vi "Write Temp YAML File.vi"(8 "Error In":errorcluster) -> (0 "Error Out":errorcluster)   [LabVIEW 2010]
panel:
  in  "Provenance":cluster{"filename":string, "software":string}={"filename"="File Name", "software"="Acquisition Software"}
  in  "Identity":T1={"author"="Author Name", "author_affiliation"="Company Name"}
  in  "Sample":T2={"sample_name"="Sample Name", "buffer_name"="Buffer Name", "dye_names"="Cy3B, ATTO647N"}
  in  "Description":string="this is a description"
  in  "Photon Data":T3={"Time Stamp Unit"=1e-08, "Measurement Type"=enum."smFRET", "Spectral Channels List"=[{"Detector IDs"=[0]}, {"Detector IDs"=[1]}]}
  in  "Excitation Types":bool[](array[boolean])=[FALSE]
  in  "detection_wavelengths":dbl[unit][](array[numeric])=[5.800000000000001e-07, 6.4e-07] caption="Detection Wavelengths"
  in  "excitation_wavelengths":dbl[unit][](array[numeric])=[5.32e-07] caption="Excitation Wavelengths"
  in  "Setup (Mandatory)":T4={"num_pixels"=2, "num_spots"=1, "num_spectral_ch"=2, "num_polarization_ch"=1, "num_split_ch"=1, "modulated_excitation"=FALSE, "lifetime"=FALSE}
  # "Photon Data"
  # "Setup (Optional)"
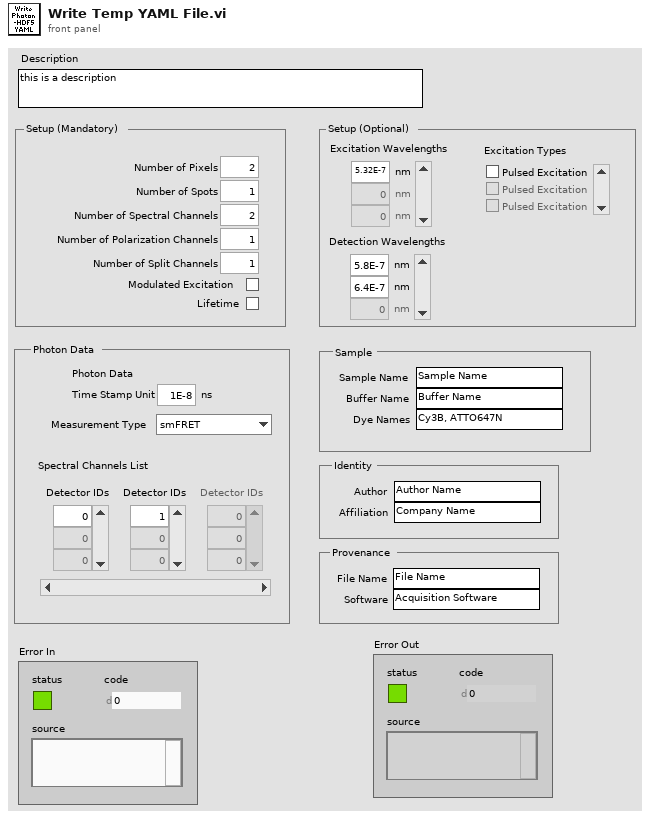
[diagram p1: front panel]
types:
  T1 = cluster{"author":string, "author_affiliation":string}
  T2 = cluster{"sample_name":string, "buffer_name":string, "dye_names":string}
  T3 = cluster{"Time Stamp Unit":dbl[unit], "Measurement Type":enum16{"Undefined", "smFRET"}, "Spectral Channels List":cluster{"Detector IDs":u8[]}[]}
  T4 = cluster{"num_pixels":u8, "num_spots":u8, "num_spectral_ch":u8, "num_polarization_ch":u8, "num_split_ch":u8, "modulated_excitation":bool, "lifetime":bool}
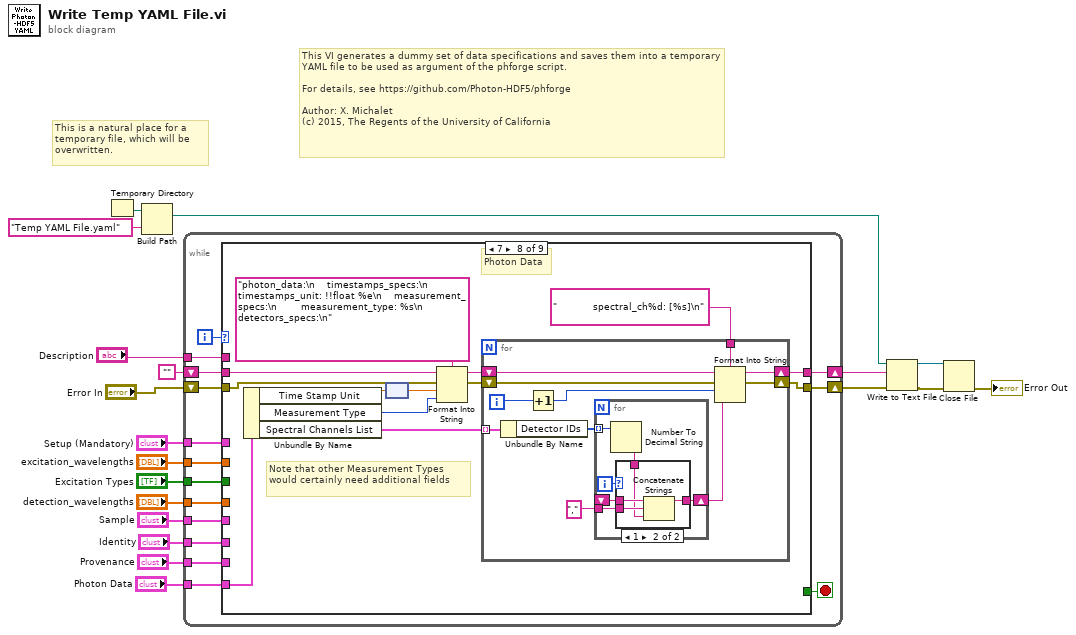
[diagram p0: block diagram]
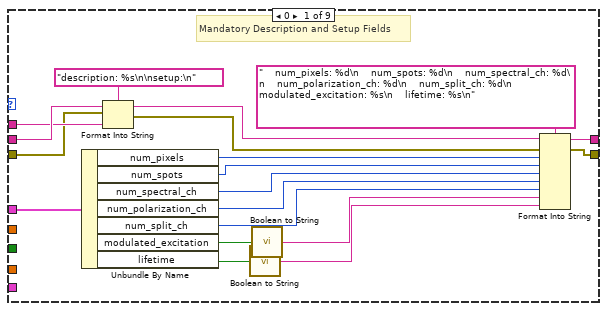
[diagram p2: hidden frame]
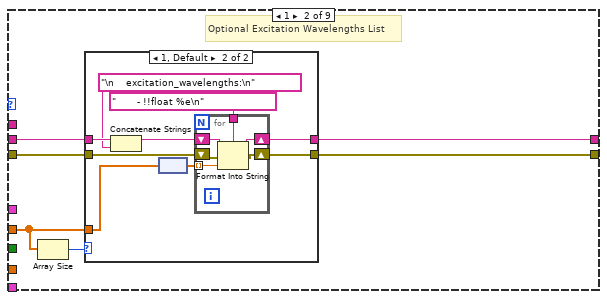
[diagram p3: hidden frame]
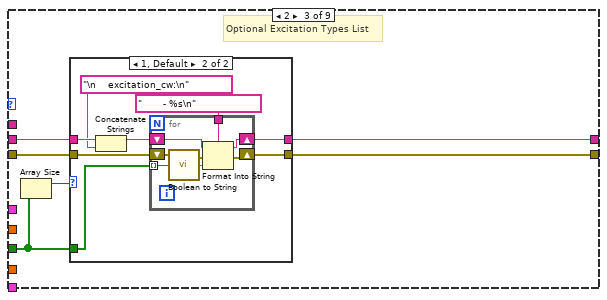
[diagram p5: hidden frame]
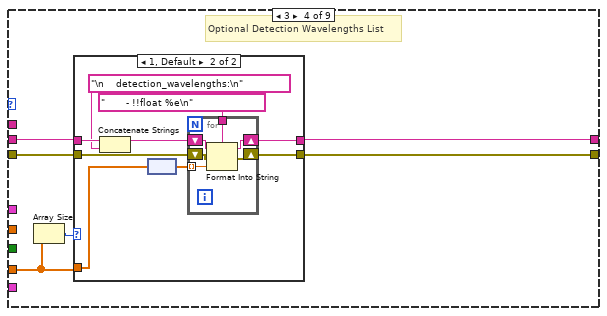
[diagram p7: hidden frame]
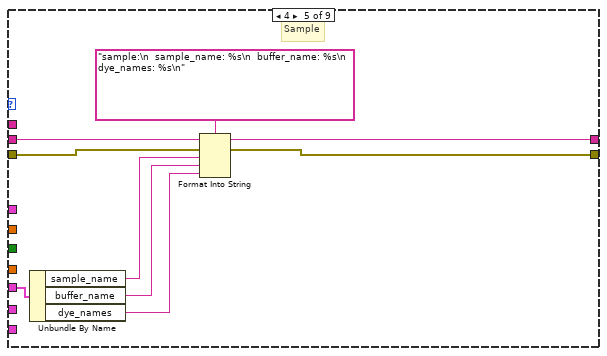
[diagram p9: hidden frame]
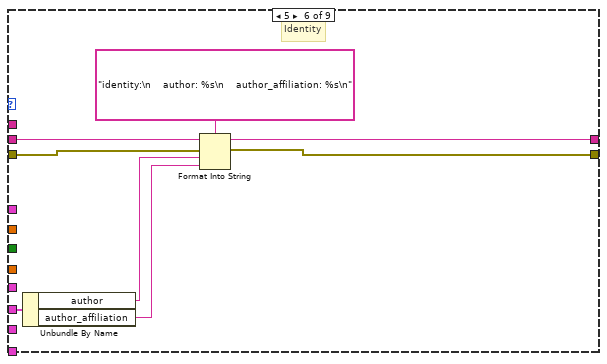
[diagram p10: hidden frame]
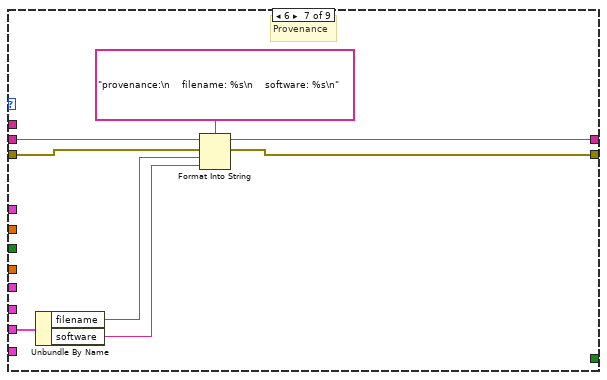
[diagram p11: hidden frame]
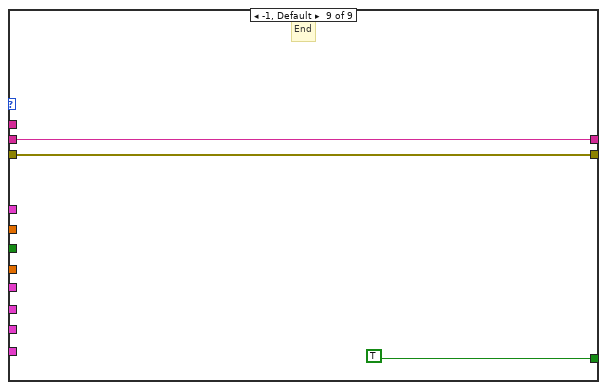
[diagram p13: hidden frame]
diagram:
  # "This is a natural place for a temporary file, which will be overwritten."
  # "This VI generates a dummy set of data specifications and saves them into a temporary YAML file to be used as argument of the phforge script.\n\nFor details, see https://github.com/Photon-HDF5/phforge\n\nAuthor: X. Michalet\n(c) 2015, The Regents of the University of California"
  n1 = Temporary Directory() -> (w14:path)
  n2 = Build Path(base path=w14, name or relative path="Temp YAML File.yaml") -> (appended path=w12:path)
  n3 = while {
    tunnel: "Setup (Mandatory)" -> [w34]
    tunnel: "excitation_wavelengths" -> [w33]
    tunnel: "Excitation Types" -> [w32]
    tunnel: "detection_wavelengths" -> [w31]
    shift-right: [w29] -> w15
    shift-left: "" -> [w30]
    tunnel: "Sample" -> [w26]
    tunnel: "Identity" -> [w25]
    tunnel: "Provenance" -> [w24]
    tunnel: "Photon Data" -> [w23]
    shift-right: [w21] -> w3
    shift-left: "Error In" -> [w22]
    tunnel: "Description" -> [w20]
    i -> [w27]
    stop <- w28 stop-if-true
    n4 = case shown="7" w27 {
      tunnel: w34 -> [w53 _ _ _ _ _ _ _ _]
      tunnel: w33 -> [_ w58 _ _ _ _ _ _ _]
      tunnel: w32 -> [_ _ w81 _ _ _ _ _ _]
      tunnel: w31 -> [_ _ _ w105 _ _ _ _ _]
      tunnel: w30 -> [w39 w56 w79 w103 w130 w139 w147 w159 w184]
      tunnel: [w44 w57 w80 w102 w126 w135 w143 w149 w184] -> w29
      tunnel: [_ _ _ _ _ _ _ _ TRUE] -> w28
      tunnel: w26 -> [_ _ _ _ w131 _ _ _ _]
      tunnel: w25 -> [_ _ _ _ _ w134 _ _ _]
      tunnel: w24 -> [_ _ _ _ _ _ w142 _ _]
      tunnel: w23 -> [_ _ _ _ _ _ _ w158 _]
      tunnel: w22 -> [w36 w54 w78 w101 w125 w133 w141 w152 w183]
      tunnel: [w43 w55 w77 w100 w124 w132 w140 w150 w183] -> w21
      tunnel: w20 -> [w38 _ _ _ _ _ _ _ _]
      frame 0 {
        # "Mandatory Description and Setup Fields"
        n5 = Unbundle By Name(w53) -> ("num_pixels"=w52:u8, "num_spots"=w51:u8, "num_spectral_ch"=w50:u8, "num_polarization_ch"=w49:u8, "num_split_ch"=w48:u8, "modulated_excitation"=w47:bool, "lifetime"=w46:bool)
        n6 = Format Into String(format string="description: %s\n\nsetup:\n", initial string=w39, error in=w36, w38) -> (resulting string=w37:string, error out=w35:errorcluster)
        n7 = call "Boolean to String.vi"("Boolean"=w46) -> ("Boolean String"=w41:string)  [unwired: 14 in]
        n8 = call "Boolean to String.vi"("Boolean"=w47) -> ("Boolean String"=w42:string)  [unwired: 14 in]
        n9 = Format Into String(format string="    num_pixels: %d\n    num_spots: %d\n    num_spectral_ch: %d\n    num_polarization_ch: %d\n    num_split_ch: %d\n    modulated_excitation: %s\n    lifetime: %s\n", initial string=w37, error in=w35, w52, w51, w50, w49, w48, w42, w41) -> (resulting string=w44:string, error out=w43:errorcluster)
      }
      frame 1 {
        # "Optional Excitation Wavelengths List"
        n10 = Array Size(array=w58) -> (size(s)=w59:i32)
        n11 = case shown="1, Default" w59 {
          tunnel: w58 -> [_ w69]
          tunnel: w56 -> [w61 w67]
          tunnel: [w61 w64] -> w57
          tunnel: [w60 w63] -> w55
          tunnel: w54 -> [w60 w62]
          frame 0 {
          }
          frame 1, Default {
            n12 = Concatenate Strings(w67, "\n    excitation_wavelengths:\n" ("string")) -> (w65:string)
            n13 = node(w69) -> (w68:dbl[])
            n14 = for {
              shift-right: [w75] -> w64
              shift-left: w65 -> [w76]
              tunnel: "       - !!float %e\n" ("resulting string") -> [w74]
              tunnel: w68 -> [w73] mode=indexing
              shift-right: [w72] -> w63
              shift-left: w62 -> [w71]
              n15 = Format Into String(format string=w74, initial string=w76, error in=w71, w73) -> (resulting string=w75:string, error out=w72:errorcluster)
            }
          }
        }
      }
      frame 2 {
        # "Optional Excitation Types List"
        n16 = Array Size(array=w81) -> (size(s)=w82:i32)
        n17 = case shown="1, Default" w82 {
          tunnel: w81 -> [_ w91]
          tunnel: w79 -> [w84 w90]
          tunnel: [w84 w87] -> w80
          tunnel: w78 -> [w83 w86]
          tunnel: [w83 w85] -> w77
          frame 0 {
          }
          frame 1, Default {
            n18 = Concatenate Strings(w90, "\n    excitation_cw:\n" ("string")) -> (w88:string)
            n19 = for {
              shift-right: [w98] -> w87
              shift-left: w88 -> [w99]
              tunnel: "       - %s\n" ("resulting string") -> [w97]
              tunnel: w91 -> [w96] mode=indexing
              shift-right: [w94] -> w85
              shift-left: w86 -> [w95]
              n20 = call "Boolean to String.vi"("Boolean"=w96) -> ("Boolean String"=w93:string)  [unwired: 14 in]
              n21 = Format Into String(format string=w97, initial string=w99, error in=w95, w93) -> (resulting string=w98:string, error out=w94:errorcluster)
            }
          }
        }
      }
      frame 3 {
        # "Optional Detection Wavelengths List"
        n22 = Array Size(array=w105) -> (size(s)=w104:i32)
        n23 = case shown="1, Default" w104 {
          tunnel: w105 -> [_ w115]
          tunnel: w103 -> [w107 w113]
          tunnel: [w107 w110] -> w102
          tunnel: w101 -> [w106 w109]
          tunnel: [w106 w108] -> w100
          frame 0 {
          }
          frame 1, Default {
            n24 = Concatenate Strings(w113, "\n    detection_wavelengths:\n" ("string")) -> (w111:string)
            n25 = node(w115) -> (w114:dbl[])
            n26 = for {
              shift-right: [w121] -> w110
              shift-left: w111 -> [w122]
              tunnel: "       - !!float %e\n" ("resulting string") -> [w120]
              tunnel: w114 -> [w119] mode=indexing
              shift-right: [w117] -> w108
              shift-left: w109 -> [w118]
              n27 = Format Into String(format string=w120, initial string=w122, error in=w118, w119) -> (resulting string=w121:string, error out=w117:errorcluster)
            }
          }
        }
      }
      frame 4 {
        # "Sample"
        n28 = Unbundle By Name(w131) -> ("sample_name"=w129:string, "buffer_name"=w128:string, "dye_names"=w123:string)
        n29 = Format Into String(format string="sample:\n  sample_name: %s\n  buffer_name: %s\n  dye_names: %s\n", initial string=w130, error in=w125, w129, w128, w123) -> (resulting string=w126:string, error out=w124:errorcluster)
      }
      frame 5 {
        # "Identity"
        n30 = Unbundle By Name(w134) -> ("author"=w138:string, "author_affiliation"=w137:string)
        n31 = Format Into String(format string="identity:\n    author: %s\n    author_affiliation: %s\n", initial string=w139, error in=w133, w138, w137) -> (resulting string=w135:string, error out=w132:errorcluster)
      }
      frame 6 {
        # "Provenance"
        n32 = Unbundle By Name(w142) -> ("filename"=w146:string, "software"=w145:string)
        n33 = Format Into String(format string="provenance:\n    filename: %s\n    software: %s\n", initial string=w147, error in=w141, w146, w145) -> (resulting string=w143:string, error out=w140:errorcluster)
      }
      frame 7 {
        # "Note that other Measurement Types would certainly need additional fields"
        # "Photon Data"
        n34 = Unbundle By Name(w158) -> ("Time Stamp Unit"=w157:dbl[unit], "Measurement Type"=w155:enum16{"Undefined", "smFRET"}, "Spectral Channels List"=w154:cluster{"Detector IDs":u8[]}[])
        n35 = node(w157) -> (w156:dbl)
        n36 = Format Into String(format string="photon_data:\n    timestamps_specs:\n        timestamps_unit: !!float %e\n    measurement_specs:\n        measurement_type: %s\n        detectors_specs:\n", initial string=w159, error in=w152, w156, w155) -> (resulting string=w153:string, error out=w151:errorcluster)
        n37 = for {
          tunnel: w154 -> [w171] mode=indexing
          shift-right: [w165] -> w149
          shift-left: w153 -> [w170]
          shift-right: [w166] -> w150
          shift-left: w151 -> [w169]
          tunnel: "            spectral_ch%d: [%s]\n" ("format string") -> [w164]
          i -> [w168]
          n38 = Unbundle By Name(w171) -> ("Detector IDs"=w163:u8[])
          n39 = Increment(x=w168) -> (x+1=w167:i32)
          n40 = for {
            tunnel: w163 -> [w177] mode=indexing
            shift-right: [w173] -> w162
            shift-left: _ -> [w175]
            tunnel: "," ("delimiter (Tab)") -> [w172]
            i -> [w176]
            n41 = Number To Decimal String(number=w177) -> (decimal integer string=w174:string)  [unwired: 1 in]
            n42 = case shown="1" w176 {
              tunnel: w175 -> [_ w182]
              tunnel: w174 -> [w178 w180]
              tunnel: [w178 w179] -> w173
              tunnel: w172 -> [_ w181]
              frame 0, Default {
              }
              frame 1 {
                n43 = Concatenate Strings(w182, w181, w180) -> (w179:string)
              }
            }
          }
          n44 = Format Into String(format string=w164, initial string=w170, error in=w169, w167, w162) -> (resulting string=w165:string, error out=w166:errorcluster)
        }
      }
      frame -1, Default {
        # "End"
      }
    }
  }
  n45 = Write to Text File(file (use dialog)=w12, text=w15, error in=w3) -> (refnum out=w9:refnum<file>, error out=w11:errorcluster)  [unwired: 1 in, 1 out]
  n46 = Close File(refnum=w9, error in=w11) -> (error out=→"Error Out":errorcluster)  [unwired: 1 out]
